vi "format.vi"(4 "Rating":refnum<vi>, 6 "Time":refnum<vi>, 7 "washData":refnum<vi>, 9 "Date":refnum<vi>, 10 "Type":refnum<vi>, 11 "washBytes":refnum<vi>) -> ()   [LabVIEW 2021]
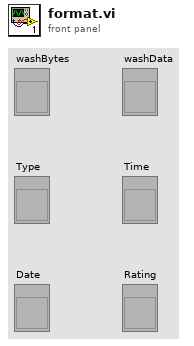
[diagram p1: front panel]
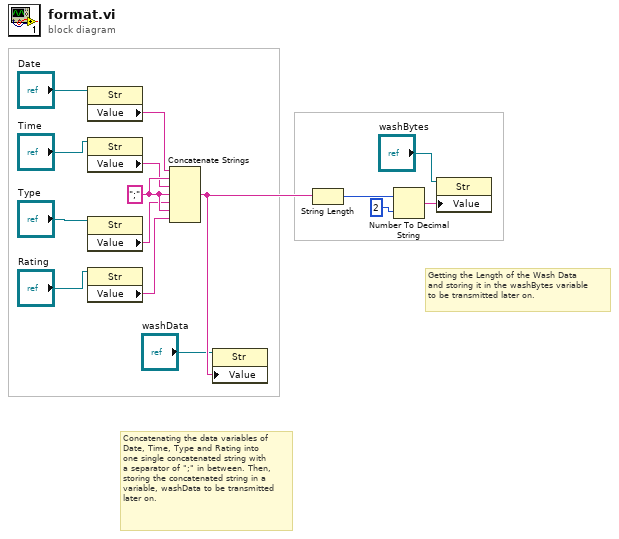
[diagram p0: block diagram]
diagram:
  w11 = ";"
  # "Concatenating the data variables of\nDate, Time, Type and Rating into\none single concatenated string with\na separator of \";\" in between. Then,\nstoring the concatenated string in a\nvariable, washData to be transmitted\nlater on."
  # "Getting the Length of the Wash Data\nand storing it in the washBytes variable\nto be transmitted later on."
  n1 = property class="Str"(reference="Date") -> ("Value"=w7:string)  [unwired: 1 in, 2 out]
  n2 = property class="Str"(reference="Time") -> ("Value"=w8:string)  [unwired: 1 in, 2 out]
  n3 = property class="Str"(reference="Type") -> ("Value"=w9:string)  [unwired: 1 in, 2 out]
  n4 = property class="Str"(reference="Rating") -> ("Value"=w10:string)  [unwired: 1 in, 2 out]
  n5 = Concatenate Strings(w7, w11, w8, w11, w9, w11, w10) -> (w14:string)
  n6 = property class="Str"(reference="washData", "Value"=w14) -> ()  [unwired: 1 in, 2 out]
  n7 = String Length(string=w14) -> (length=w12:i32)
  n8 = Number To Decimal String(number=w12, width (-)=i16 2) -> (decimal integer string=w13:string)
  n9 = property class="Str"(reference="washBytes", "Value"=w13) -> ()  [unwired: 1 in, 2 out]
